vi "cast_boolean_notifier.vi"   [LabVIEW 2015]
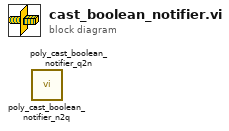
[diagram p0: block diagram]
diagram:
  n1 = call "poly_cast_boolean_notifier_n2q.vi"() -> ()  [unwired: 9 in, 1 out]
  n2 = call "poly_cast_boolean_notifier_q2n.vi"() -> ()  [unwired: 9 in, 1 out]
